vi "Form GLL Sentence.vi"(8 "error in (no error)":errorcluster, 11 "GLL data":T1={"latitude"={"included?"=TRUE, "latitude (deg)"=0.0}, "longitude"={"included?"=TRUE, "longitude (deg)"=0.0}, "time of fix"={"included?"=TRUE, "time (UTC)"=timestamp(1451718000 s since 1904-01-01)}, "status"={"included?"=TRUE, "value"=0}, "type of fix"={"included?"=TRUE, "mode"=0}} {"type of fix"."mode" items=["Simulator", "Not Valid", "Estimated", "Differential", "Autonomous"]; "status"."value" items=["Void", "Active"]; "time of fix"."time (UTC)" format="%^<%.3X\n%x>T"}) -> (0 "error out":errorcluster, 3 "GLL sentence":string)   [LabVIEW 2017, in "NMEA API.lvlib"]
doc: "Creates an NMEA sentence using the data you specify for a particular sentence type. You must manually select the polymorphic instance to use."
uses:
  <vilib>/robotics/Protocols/NMEA/NMEA API.lvlib
  <vilib>/robotics/Protocols/NMEA/typedefs/GLL Data.ctl
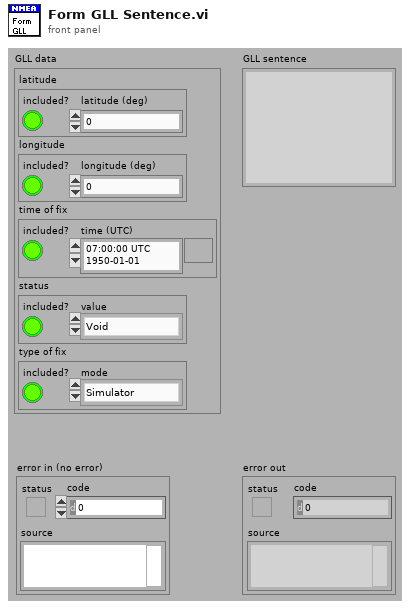
[diagram p1: front panel]
types:
  T1 = typedef "NMEA API.lvlib/GLL Data.ctl" = cluster{"latitude":cluster{"included?":bool, "latitude (deg)":dbl}, "longitude":cluster{"included?":bool, "longitude (deg)":dbl}, "time of fix":cluster{"included?":bool, "time (UTC)":timestamp}, "status":cluster{"included?":bool, "value":u16}, "type of fix":cluster{"included?":bool, "mode":u16}}
  T2 = cluster{"included?":bool, "time (UTC)":timestamp}
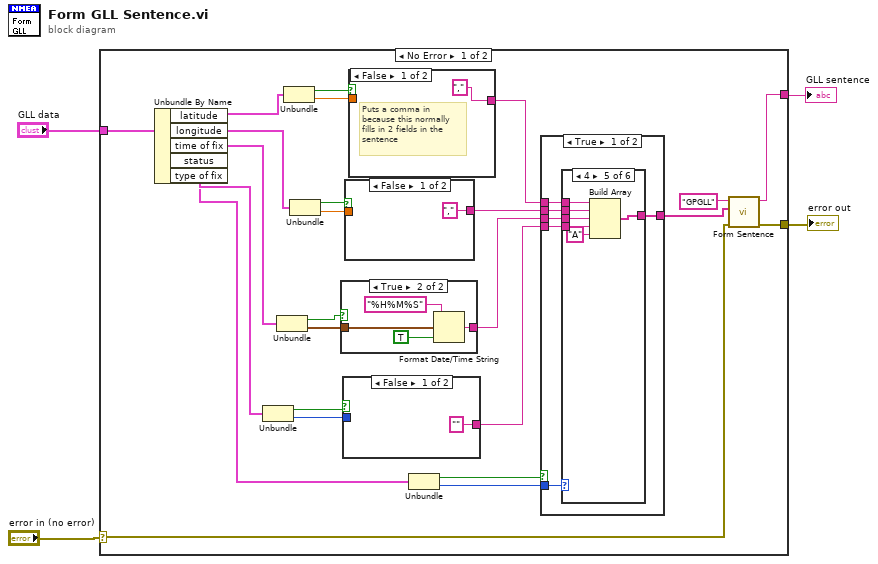
[diagram p0: block diagram]
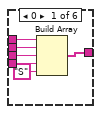
[diagram p2: hidden frame]
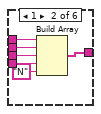
[diagram p3: hidden frame]
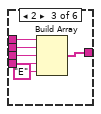
[diagram p4: hidden frame]
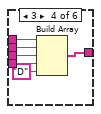
[diagram p5: hidden frame]
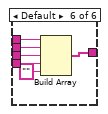
[diagram p6: hidden frame]
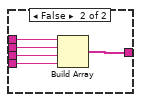
[diagram p7: hidden frame]
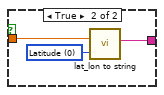
[diagram p8: hidden frame]
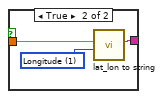
[diagram p9: hidden frame]
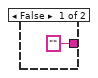
[diagram p10: hidden frame]
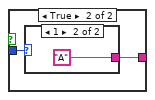
[diagram p11: hidden frame]
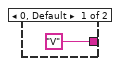
[diagram p12: hidden frame]
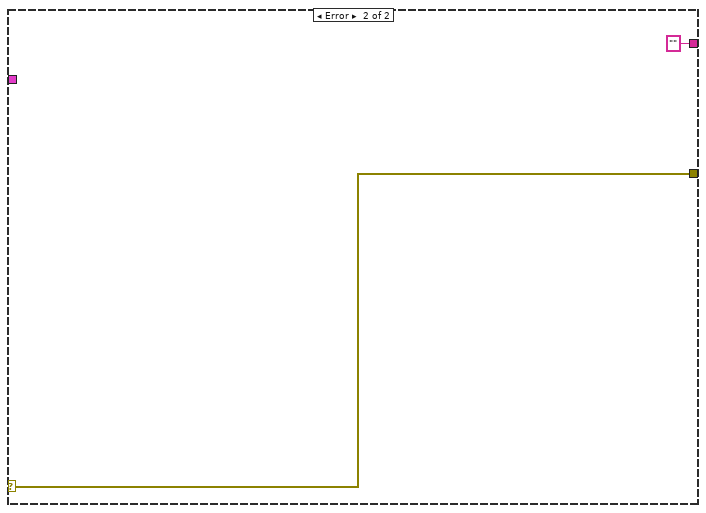
[diagram p13: hidden frame]
diagram:
  n1 = case shown="No Error" "error in (no error)" {
    selector: "error in (no error)" -> [w8 w95]
    tunnel: "GLL data" -> [w29 _]
    tunnel: [w26 w95] -> w2
    tunnel: [w25 "" ("NMEA Sentence")] -> w1
    frame No Error {
      n2 = Unbundle By Name(w29) -> ("latitude"=w20:cluster{"included?":bool, "latitude (deg)":dbl}, "longitude"=w18:cluster{"included?":bool, "longitude (deg)":dbl}, "time of fix"=w16:T2, "status"=w14:cluster{"included?":bool, "value":u16}, "type of fix"=w7:cluster{"included?":bool, "mode":u16})
      n3 = Unbundle(w14) -> ("included?"=w12:bool, "value"=w13:u16)
      n4 = Unbundle(w16) -> ("included?"=w11:bool, "time (UTC)"=w15:timestamp)
      n5 = Unbundle(w20) -> ("included?"=w9:bool, "latitude (deg)"=w19:dbl)
      n6 = Unbundle(w18) -> ("included?"=w10:bool, "longitude (deg)"=w17:dbl)
      n7 = case shown="True" w11 {
        tunnel: ["" ("date/time string") w88] -> w24
        tunnel: w15 -> [_ w87]
        frame False {
        }
        frame True {
          n8 = Format Date/Time String(time format string (%c)="%H%M%S", seconds (now)=w87, UTC format=TRUE) -> (date/time string=w88:string)
        }
      }
      n9 = case shown="False" w12 {
        tunnel: ["" w92] -> w23
        tunnel: w13 -> [_ w91]
        frame False {
        }
        frame True {
          n10 = case shown="1" w91 {
            tunnel: ["V" "A"] -> w92
            frame 0, Default {
            }
            frame 1 {
            }
          }
        }
      }
      n11 = case shown="False" w10 {
        tunnel: ["," ("NMEA String for Lat/Lon") w83] -> w21
        tunnel: w17 -> [_ w82]
        frame False {
        }
        frame True {
          w84 = u16 1 items=["Latitude", "Longitude"] ("Lat/Lon")
          n12 = call <vilib>:"lat_lon to string.vi"("lat/lon"=w84, "composite value"=w82) -> ("NMEA string for lat/lon"=w83:string)  [unwired: 9 out]
        }
      }
      n13 = case shown="False" w9 {
        tunnel: ["," ("NMEA String for Lat/Lon") w79] -> w22
        tunnel: w19 -> [_ w78]
        frame False {
          # "Puts a comma in\nbecause this normally\nfills in 2 fields in the \nsentence"
        }
        frame True {
          w80 = u16 0 items=["Latitude", "Longitude"] ("Lat/Lon")
          n14 = call <vilib>:"lat_lon to string.vi"("lat/lon"=w80, "composite value"=w78) -> ("NMEA string for lat/lon"=w79:string)  [unwired: 9 out]
        }
      }
      n15 = Unbundle(w7) -> ("included?"=w6:bool, "mode"=w5:u16)
      n16 = case shown="True" w6 {
        tunnel: [w35 w76] -> w27
        tunnel: w24 -> [w34 w75]
        tunnel: w23 -> [w33 w74]
        tunnel: w22 -> [w32 w73]
        tunnel: w21 -> [w31 w72]
        tunnel: w5 -> [w30 _]
        frame True {
          n17 = case shown="4" w30 {
            tunnel: [w41 w47 w53 w59 w65 w71] -> w35
            tunnel: w34 -> [w40 w46 w52 w58 w64 w70]
            tunnel: w33 -> [w39 w45 w51 w57 w63 w69]
            tunnel: w32 -> [w38 w44 w50 w56 w62 w68]
            tunnel: w31 -> [w37 w43 w49 w55 w61 w67]
            frame 0 {
              n18 = Build Array(w38, w37, w40, w39, "S" ("element")) -> (w41:string[])
            }
            frame 1 {
              n19 = Build Array(w44, w43, w46, w45, "N" ("element")) -> (w47:string[])
            }
            frame 2 {
              n20 = Build Array(w50, w49, w52, w51, "E" ("element")) -> (w53:string[])
            }
            frame 3 {
              n21 = Build Array(w56, w55, w58, w57, "D" ("element")) -> (w59:string[])
            }
            frame 4 {
              n22 = Build Array(w62, w61, w64, w63, "A" ("element")) -> (w65:string[])
            }
            frame Default {
              n23 = Build Array(w68, w67, w70, w69, "" ("element")) -> (w71:string[])
            }
          }
        }
        frame False {
          n24 = Build Array(w73, w72, w75, w74) -> (w76:string[])
        }
      }
      n25 = call <vilib>:"Form Sentence.vi"("error in (no error)"=w8, "sentence data"=w27, "sentence type"="GPGLL" ("Sentence Type")) -> ("error out"=w26:errorcluster, "sentence"=w25:string)  [unwired: 5 in]
    }
    frame Error {
    }
  }
  "error out" <- w2
  "GLL sentence" <- w1
